vi "Archive Directories.vi"(8 "Error In":errorcluster, 9 "Archive Dest":path=path "C:/Program Files/National Instruments/LabVIEW 2013/vi.lib/LabVIEW Hacker/EZ430-Chronos-Interface-bak.zip", 10 "Archive Root":path=path "C:/Program Files/National Instruments/LabVIEW 2013", 11 "Directory Paths":path[](array[path])=[path "C:/Program Files/National Instruments/LabVIEW 2013/vi.lib/LabVIEW Hacker/EZ430-Chronos-Interface", path "C:/Program Files/National Instruments/LabVIEW 2013/examples/LabVIEW Hacker/EZ430-Chronos-Interface", path "C:/Program Files/National Instruments/LabVIEW 2013/examples/exbins/LabVIEW Hacker/EZ430-Chronos-Interface", path "C:/Program Files/National Instruments/LabVIEW 2013/menus/Categories/EZ430-Chronos"]) -> (0 "Error Out":errorcluster)   [LabVIEW 2011, in "LMH-Toolbox.lvlib"]
doc: "Build archive containing multiple folders. Archive Root is a parent folder common to all Directory Paths. All files are stored in the archive relative to archive root."
uses:
  LMH-Toolbox.lvlib
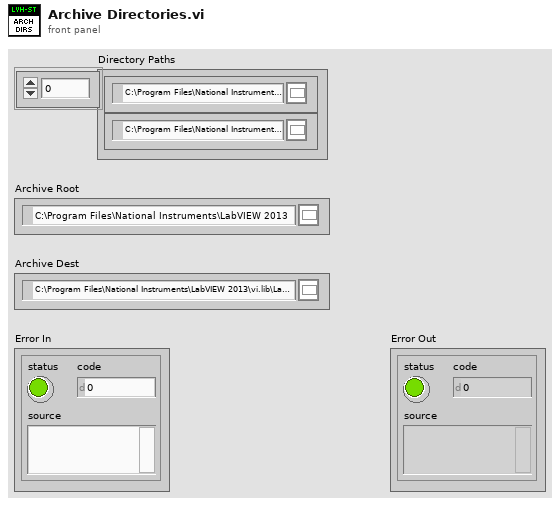
[diagram p1: front panel]
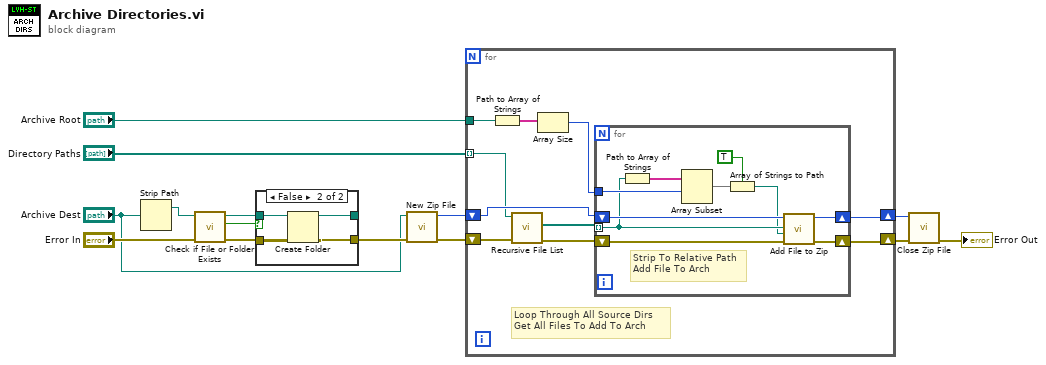
[diagram p0: block diagram]
diagram:
  n1 = Strip Path(path="Archive Dest") -> (stripped path=w2:path)  [unwired: 1 out]
  n2 = call <vilib>:"Check if File or Folder Exists.vi"("error in (no error)"="Error In", "path"=w2) -> ("error out"=w6:errorcluster, "file or folder exists?"=w7:bool, "dup path"=w3:path)  [unwired: 7 in]
  n3 = case shown="False" w7 {
    tunnel: w3 -> [w15 w18]
    tunnel: [w16 w19] -> w4
    tunnel: w6 -> [w16 w20]
    tunnel: [w15 w17] -> _
    frame True {
    }
    frame False {
      n4 = Create Folder(path (use dialog)=w18, error in=w20) -> (created path=w17:path, error out=w19:errorcluster)  [unwired: 1 in, 1 out]
    }
  }
  n5 = call <vilib>:"New Zip File.vi"("error in (no error)"=w4, "target"="Archive Dest") -> ("error out"=w10:errorcluster, "zip file out"=w13:i64)  [unwired: 3 in, 1 out]
  n6 = for {
    tunnel: "Directory Paths" -> [w22] mode=indexing
    shift-right: [w28] -> w12
    shift-left: w10 -> [w24]
    shift-right: [w27] -> w11
    shift-left: w13 -> [w29]
    tunnel: "Archive Root" -> [w21]
    # "Loop Through All Source Dirs\nGet All Files To Add To Arch"
    n7 = Path to Array of Strings(0:w21) -> (2:w26:string[])  [unwired: 1 out]
    n8 = call <vilib>:"Recursive File List.vi"("error in (no error)"=w24, "Folder Path"=w22) -> ("error out"=w23:errorcluster, "All Files in Dir"=w30:path[])  [unwired: 5 in, 3 out]
    n9 = Array Size(array=w26) -> (size(s)=w25:i32)
    n10 = for {
      tunnel: w30 -> [w32] mode=indexing
      shift-right: [w37] -> w28
      shift-left: w23 -> [w39]
      shift-right: [w38] -> w27
      shift-left: w29 -> [w40]
      tunnel: w25 -> [w33]
      # "Strip To Relative Path\nAdd File To Arch"
      n11 = Path to Array of Strings(0:w32) -> (2:w36:string[])  [unwired: 1 out]
      n12 = Array Subset(array=w36, index=w33) -> (w35:string[])  [unwired: 1 in]
      n13 = Array of Strings to Path(0:w35, 1:TRUE ("relative")) -> (2:w31:path)
      n14 = call <vilib>:"Add File to Zip.vi"("error in (no error)"=w39, "destination path in zip"=w31, "source file path"=w32, "zip file in"=w40) -> ("error out"=w37:errorcluster, "zip file out"=w38:i64)  [unwired: 6 in]
    }
  }
  n15 = call <vilib>:"Close Zip File.vi"("error in (no error)"=w12, "zip file in"=w11) -> ("error out"=→"Error Out":errorcluster)  [unwired: 5 in]
